vi "TEST ALL.vi"(8 "error in":errorcluster) -> (0 "error out":errorcluster)   [LabVIEW 2017]
uses:
  <vilib>/addons/_JKI Toolkits/Caraya/classes/Test/Test.lvclass
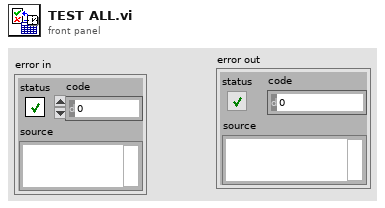
[diagram p1: front panel]
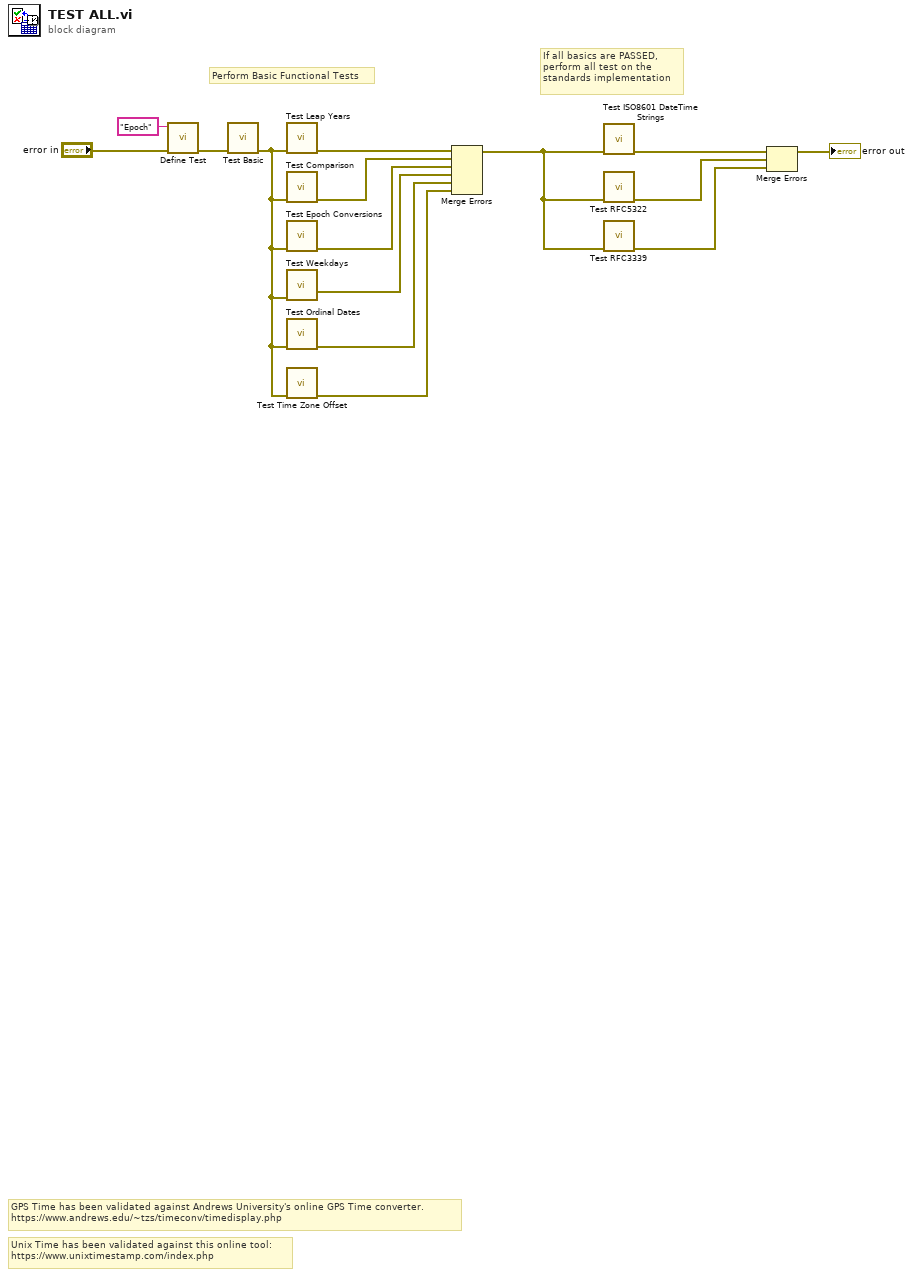
[diagram p0: block diagram]
diagram:
  # "If all basics are PASSED, \nperform all test on the \nstandards implementation"
  # "Perform Basic Functional Tests"
  # "Unix Time has been validated against this online tool:\nhttps://www.unixtimestamp.com/index.php"
  # "GPS Time has been validated against Andrews University's online GPS Time converter.\nhttps://www.andrews.edu/~tzs/timeconv/timedisplay.php"
  n1 = call <vilib>:"Define Test.vi"("error in (no error)"="error in", "Label (VI Title)"="Epoch") -> ("error out"=w14:errorcluster)  [unwired: 8 in, 1 out]
  n2 = call "Test Basic.vi"("error in"=w14) -> ("error out"=w2:errorcluster)  [unwired: 10 in]
  n3 = call "Test Leap Years.vi"("error in"=w2) -> ("error out"=w12:errorcluster)  [unwired: 10 in]
  n4 = call "Test Comparison.vi"("error in"=w2) -> ("error out"=w13:errorcluster)  [unwired: 10 in]
  n5 = call "Test Epoch Conversions.vi"("error in"=w2) -> ("error out"=w11:errorcluster)  [unwired: 10 in]
  n6 = call "Test Weekdays.vi"("error in"=w2) -> ("error out"=w10:errorcluster)  [unwired: 10 in]
  n7 = call "Test Ordinal Dates.vi"("error in"=w2) -> ("error out"=w9:errorcluster)  [unwired: 10 in]
  n8 = call "Test Time Zone Offset.vi"("error in"=w2) -> ("error out"=w1:errorcluster)  [unwired: 10 in]
  n9 = Merge Errors(w12, w13, w11, w10, w9, w1) -> (w4:errorcluster)
  n10 = call "Test ISO8601 DateTime Strings.vi"("error in"=w4) -> ("error out"=w7:errorcluster)  [unwired: 10 in]
  n11 = call "Test RFC5322.vi"("error in"=w4) -> ("error out"=w5:errorcluster)  [unwired: 10 in]
  n12 = call "Test RFC3339.vi"("error in"=w4) -> ("error out"=w3:errorcluster)  [unwired: 10 in]
  n13 = Merge Errors(w7, w5, w3) -> (→"error out":errorcluster)
